vi "FXP LMS.vi"(7 "reset? (F)":bool, 9 "step size":fxp<+/-,16,-1>=0.01000213623046875, 10 "d(n)":fxp<+/-,24,4>, 11 "x(n)":fxp<+/-,24,4>) -> (0 "coefficients overflow":bool, 2 "e(n)":fxp<+/-,24,4>, 3 "y(n)":fxp<+/-,24,4>)   [LabVIEW 2019]
doc: "Contains the settings of a fixed-point LMS adaptive filter.\n\nThis VI is configured as follows:\n\nFilter length: 1000\nDefault step size: 1.000214E-2\n\nx(n) word length: 24\nx(n) integer word length: 4\n\nd(n) word length: 24\nd(n) integer word length: 4\n\nw(n) word length: 24\nw(n) integer word length: 4\n\nstep size word length: 16\nstep size integer word length: -1\n\nThe data type of e(n) and y(n) is the same as that of d(n).\n\nTo change the settings of this fixed-point LMS adaptive filter, you must generate LabVIEW FPGA code for this filter again."
uses:
  <vilib>/Platform/TimedLoop/XDataNode/timing_clust.ctl
  <vilib>/Platform/TimedLoop/XDataNode/nitl_modes.ctl
  <vilib>/Platform/TimedLoop/XDataNode/wakeup.ctl
  <vilib>/rvi/DataTransferAndStorage/Container/Common/niFpgaContainerGetUniqueNameForEmu.vi
  <vilib>/rvi/DataTransferAndStorage/Container/Common/niFpgaContainerSetEmuInfo.vi
  <vilib>/rvi/eio/common/nirviEmuReportErrorAndStop.vi
  <vilib>/rvi/Emulation/niFpgaSctlEmulationGetInTimedLoop.vi
  <vilib>/rvi/Emulation/niFpgaEmulationReportErrorSimple.vi
  <vilib>/rvi/Emulation/niFpgaGetClockAttributes.vi
  <vilib>/rvi/Emulation/niFpgaCriticalErrorInLSC.vi
  <vilib>/rvi/Memory/Memory_Emulation/nirvimemoryEmulation.vi
  <vilib>/rvi/Memory/Memory_Emulation/nirvimemoryFastEmulation.vi
  <vilib>/rvi/Memory/Memory_Emulation/niFpgaMemoryEmulationCacheClearOnFirstRun.vi
  <vilib>/rvi/Memory/Memory_Emulation/nirvimemoryEmulationManagerCache_MakeExclusive.vi
  <vilib>/rvi/Memory/Memory_Emulation/niFpgaMemoryEmulationValidateCache.vi
  <vilib>/rvi/Memory/Memory_Emulation/nirvimemoryEmulationManagerCache_InsertValue.vi
  <vilib>/Utility/error.llb/Clear Errors.vi
  <vilib>/rvi/Memory/Memory_Emulation/nirvimemoryEmulationManagerCache_ReleaseExclusive.vi
  <vilib>/rvi/Memory/Memory_Emulation/nirvimemoryEmulationManagerCache_GetValue.vi
  <vilib>/rvi/Emulation/niFpgaEmulationIsFPGAContextNoSignature.vi
  <vilib>/rvi/Memory/Memory_Emulation/nirvimemoryEmulationManagerCache_SetValue.vi
  <vilib>/rvi/Emulation/niFpgaSctlEmulationResourceMgr.vi
  <vilib>/rvi/LocalResourceManager/LocalResourceManager.xnode
  <vilib>/Platform/TimedLoop/XDataNode/XDataNode.xnode
  <vilib>/rvi/DataTransferAndStorage/Container/XNode/niFpgaContainer.xnode
  <vilib>/rvi/FXPMathLib/FxpMul/XNode/nifxpmath_Multiplier.xnode
  <vilib>/Platform/TimedLoop/XDataNode/XDNodeRunTimeDep.lvlib
  <vilib>/rvi/FXPMathLib/sim/FxpSim.dll
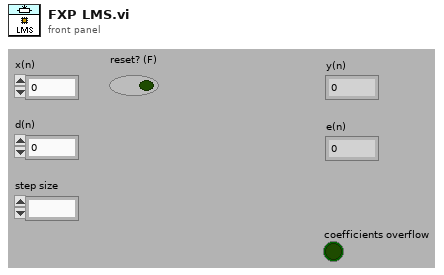
[diagram p1: front panel]
types:
  T1 = typedef "XDNodeRunTimeDep.lvlib/timing_clust.ctl" = cluster{"Expected End [f-1]":u64, "Actual End [f-1]":u64, "Finished Late? [f-1]":bool, "Expected End [i-1]":u64, "Actual End [i-1]":u64, "Finished Late? [i-1]":bool, "Expected Start [i]":u64, "Actual Start [i]":u64, "Expected Start [f]":u64, "Actual Start [f]":u64, "Source Name":string, "Structure Name":string, "Period":i64, "Deadline":i64, "Offset":i64, "Start":i64, "Priority":i32, "Timeout":i32, "Mode":T2, "Wakeup Reason":T3, "Error":errorcluster, "Source Type":string, "Secondary Source Type":string, "Global End Time":u64, "Global Start Time":u64, "Frame Duration":u64, "Iteration Duration":u64, "Assigned CPU":i32, "I/O Scan Engine Mode":u32}
  T2 = typedef "XDNodeRunTimeDep.lvlib/nitl_modes.ctl" = enum32{"No Change", "Process missed periods, maintain original phase", "Discard missed periods, maintain original phase", "Process missed periods, ignore original phase", "Discard missed periods, ignore original phase"}
  T3 = typedef "XDNodeRunTimeDep.lvlib/wakeup.ctl" = enum32{"Normal", "Aborted", "Asynchronous wakeup", "Timing source error", "Timed loop error", "Timeout"}
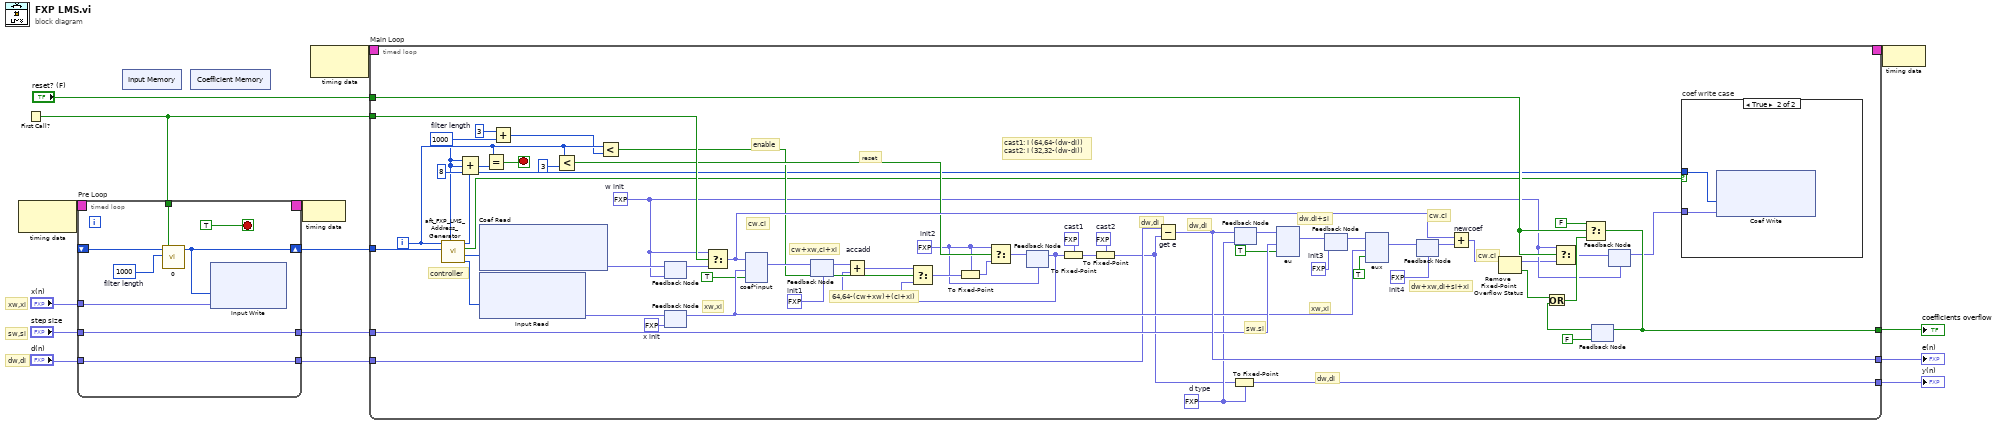
[diagram p0: block diagram]
diagram:
  # "dw,di"
  # "sw,si"
  # "xw,xi"
  n1 = node-c288() -> (w2:T1)  [unwired: 1 in]
  n2 = First Call?() -> (First Call?: T/F=w7:bool)
  n3 = timed-loop "Pre Loop" {
    tunnel: w7 -> [w18]
    shift-right: [w19] -> w15
    shift-left: _ -> [w17]
    tunnel: "x(n)" -> [w21]
    tunnel: "d(n)" -> [w20]
    tunnel: [w20] -> w12
    tunnel: "step size" -> [w22]
    tunnel: [w22] -> w9
    timing: w2 -> [_]
    timing-out: [_] -> w1
    stop <- TRUE stop-if-true
    w16 = u32 1000  # filter length
    n4 = call "0"("first run? (F)"=w18, "filter length"=w16, "state in"=w17) -> ("state out"=w19:u32)  [unwired: 8 in]
    n5 = xnode ("Input Write")("Address"=w19, "Data"=w21) -> ()  [unwired: 1 in, 1 out]
  }
  n6 = xnode "Input Memory"() -> ()  [unwired: 1 out]
  n7 = xnode "Coefficient Memory"() -> ()  [unwired: 1 out]
  n8 = node-c288(w1) -> ()
  n9 = node-c288() -> (w4:T1)  [unwired: 1 in]
  n10 = timed-loop "Main Loop" {
    tunnel: w15 -> [w84]
    tunnel: w12 -> [w30]
    tunnel: [w69] -> w11
    tunnel: w9 -> [w67]
    tunnel: [w54] -> w8
    tunnel: w7 -> [w72]
    tunnel: "reset? (F)" -> [w56]
    tunnel: [w70] -> w5
    timing: w4 -> [_]
    timing-out: [_] -> w3
    i -> [w82]
    stop <- w87 stop-if-true
    w26 = fxp<+/-,32,12> 0.0  # cast2
    w29 = fxp<+/-,64,44> 0.0  # cast1
    w45 = fxp<+/-,24,4> 0.0  # d type
    w33 = fxp<+/-,64,24> 0.0  # init2
    w75 = fxp<+/-,48,7> 0.0  # init4
    w76 = fxp<+/-,24,3> 0.0  # init3
    w77 = fxp<+/-,48,8> 0.0  # init1
    w73 = 1000  # filter length
    w48 = fxp<+/-,24,4> 0.0  # x init
    w44 = fxp<+/-,24,4> 0.0  # w init
    # "cast1: I (64,64-(dw-di))\ncast2: I (32,32-(dw-di))"
    # "cw.ci"
    # "xw,xi"
    # "dw,di"
    # "64,64-(cw+xw)+(ci+xi)"
    # "enable"
    # "reset"
    # "cw.ci"
    # "dw,di"
    # "dw+xw,di+si+xi"
    # "dw.di+si"
    # "dw,di"
    # "cw+xw,ci+xi"
    # "cw.ci"
    # "xw,xi"
    # "sw.si"
    # "controller"
    n11 = call <vilib>:"aft_FXP_LMS_Address_Generator.vi"("filter length"=w73, "initialize x read address"=w84, "index"=w82) -> ("x read address"=w85:u32, "coefficient read address"=w86:u32, "coefficient write enable"=w40:bool, "coefficient write address"=w39:u32)  [unwired: 5 out]
    n12 = Compound Arithmetic op=unknown(w73, w73, 8 ("value")) -> (w81:i32)
    n13 = xnode ("Coef Read")("Address"=w86) -> ("Data"=w47:fxp<+/-,24,4>)  [unwired: 1 in, 1 out]
    n14 = xnode ("Input Read")("Address"=w85) -> ("Data"=w46:fxp<+/-,24,4>)  [unwired: 1 in, 1 out]
    n15 = Equal?(x=w82, y=w81) -> (x = y?=w87:bool)
    n16 = Add(x=3, y=w73) -> (x+y=w78:i32)
    n17 = Less?(x=w82, y=3) -> (x < y?=w52:bool)
    n18 = Less?(x=w82, y=w78) -> (x < y?=w51:bool)
    n19 = feedback-in #1(w47) -> ()
    n20 = feedback #1(w44) -> (w74:fxp<+/-,24,4>)
    n21 = feedback-in #2(w46) -> ()
    n22 = feedback #2(w48) -> (w64:fxp<+/-,24,4>)
    n23 = Select(t=w44, s=w72, f=w74) -> (s? t:f=w61:fxp<+/-,24,4>)
    n24 = xnode "coef*input"("x"=w61, "y"=w64, "input valid"=TRUE) -> ("x*y"=w71:fxp<+/-,48,8>)  [unwired: 1 in, 2 out]
    n25 = feedback-in #3(w71) -> ()
    n26 = feedback #3(w77) -> (w50:fxp<+/-,48,8>)
    n27 = feedback #4(w33) -> (w37:fxp<+/-,64,24>)
    n28 = Add "accadd"(x=w50, y=w37) -> (x+y=w53:fxp<+/-,64,24>)
    n29 = Select(t=w53, s=w51, f=w37) -> (s? t:f=w36:fxp<+/-,64,24>)
    n30 = To Fixed-Point(fixed-point type=w33, number=w36) -> (fixed-point=w34:fxp<+/-,64,24>)
    n31 = Select(t=w33, s=w52, f=w34) -> (s? t:f=w49:fxp<+/-,64,24>)
    n32 = feedback-in #4(w49) -> ()
    n33 = To Fixed-Point(fixed-point type=w29, number=w37) -> (fixed-point=w28:fxp<+/-,64,44>)
    n34 = To Fixed-Point(fixed-point type=w26, number=w28) -> (fixed-point=w27:fxp<+/-,32,12>)
    n35 = Subtract "get e"(x=w30, y=w27) -> (x-y=w69:fxp<+/-,24,4>)
    n36 = To Fixed-Point ("2fxp")(fixed-point type=w45, number=w27) -> (fixed-point=w70:fxp<+/-,24,4>)
    n37 = feedback-in #5(w69) -> ()
    n38 = feedback #5(w45) -> (w68:fxp<+/-,24,4>)
    n39 = xnode "eu"("x"=w68, "y"=w67, "input valid"=TRUE) -> ("x*y"=w66:fxp<+/-,24,3>)  [unwired: 1 in, 2 out]
    n40 = feedback-in #6(w66) -> ()
    n41 = feedback #6(w76) -> (w65:fxp<+/-,24,3>)
    n42 = xnode "eux"("x"=w65, "y"=w64, "input valid"=TRUE) -> ("x*y"=w63:fxp<+/-,48,7>)  [unwired: 1 in, 2 out]
    n43 = feedback-in #7(w63) -> ()
    n44 = feedback #7(w75) -> (w62:fxp<+/-,48,7>)
    n45 = Add "newcoef"(x=w61, y=w62) -> (x+y=w32:fxp<+/-,24,4>)
    n46 = Remove Fixed-Point Overflow Status(3:w32) -> (0:w35:bool, 1:w31:fxp<+/-,24,4>)
    n47 = Select(t=w44, s=w56, f=w31) -> (s? t:f=w55:fxp<+/-,24,4>)
    n48 = feedback #8(FALSE ("overflow")) -> (w57:bool)
    n49 = Or(x=w35, y=w57) -> (x .or. y?=w60:bool)
    n50 = Select(t=FALSE, s=w56, f=w60) -> (s? t:f=w54:bool)
    n51 = feedback-in #8(w54) -> ()
    n52 = feedback-in #9(w55) -> ()
    n53 = feedback #9(w44) -> (w38:fxp<+/-,24,4>)
    n54 = case "coef write case" shown="True" w40 {
      tunnel: w39 -> [_ w89]
      tunnel: w38 -> [_ w88]
      frame False {
      }
      frame True {
        n55 = xnode ("Coef Write")("Address"=w89, "Data"=w88) -> ()  [unwired: 1 in, 1 out]
      }
    }
  }
  "e(n)" <- w11
  "coefficients overflow" <- w8
  "y(n)" <- w5
  n56 = node-c288(w3) -> ()
